vi "GetEnumerator.vi"(8 "Error In":errorcluster, 11 "object in":refnum<class "IEnumerable.lvclass">) -> (0 "Error Out":errorcluster, 2 "Return(LabVIEW Class)":refnum<class "IEnumerator.lvclass">, 3 "object out":refnum<class "IEnumerable.lvclass">)   [LabVIEW 2020, in "IEnumerable.lvclass"]
doc: "Interfaces are not serializable\nReturns an IEnumerator for this enumerable Object. The enumerator provides\na simple way to access all the contents of a collection."
uses:
  IEnumerable.lvclass
  IEnumerator_interface/IEnumerator.lvclass
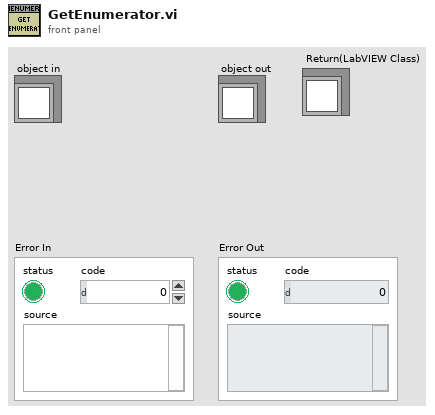
[diagram p1: front panel]
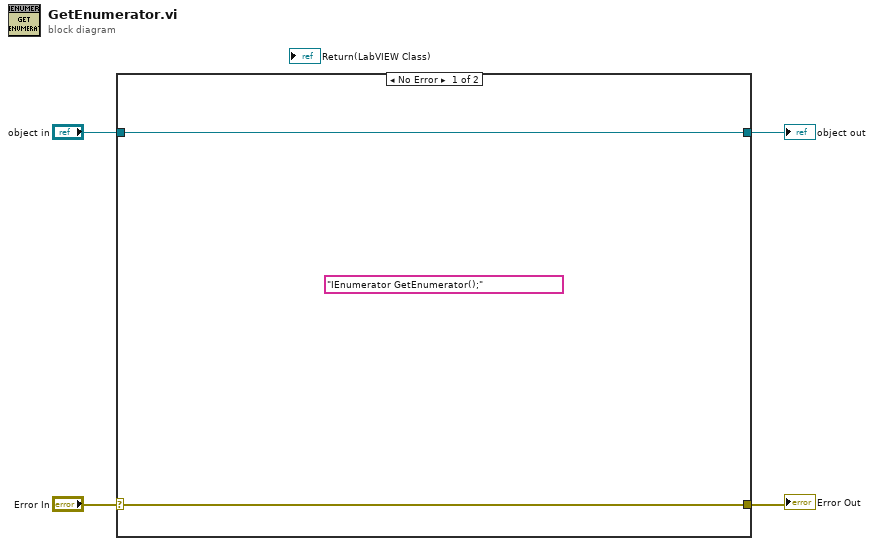
[diagram p0: block diagram]
diagram:
  (unwired) "IEnumerator GetEnumerator();"
  n1 = case shown="No Error" "Error In" {
    selector: "Error In" -> [w6 w8]
    tunnel: [w6 w8] -> w3
    tunnel: [w5 w7] -> w1
    tunnel: "object in" -> [w5 w7]
    frame No Error {
    }
    frame Error {
    }
  }
  "Error Out" <- w3
  "object out" <- w1
